vi "GetType.vi"(8 "error in (no error)":errorcluster, 11 "Configure Acceleration Msg":refnum<class "Configure Acceleration Msg.lvclass">) -> (0 "error out":errorcluster, 2 "Data Sample":variant, 3 "Configure Acceleration Msg":refnum<class "Configure Acceleration Msg.lvclass">)   [LabVIEW 2015, in "CS++Motor.lvlib" / "Configure Acceleration Msg.lvclass"]
uses:
  Configure Acceleration Msg.lvclass
  Configure Acceleration Msg.lvclass/Configure Acceleration Msg.ctl
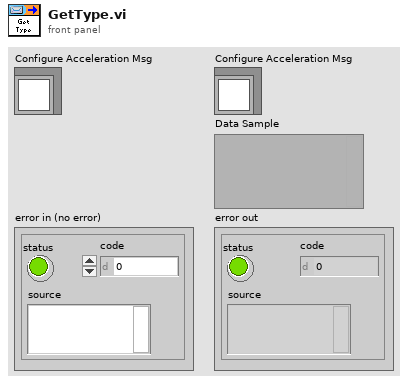
[diagram p1: front panel]
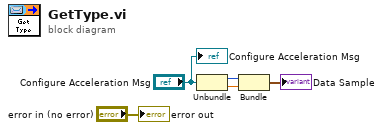
[diagram p0: block diagram]
diagram:
  n1 = Unbundle("Configure Acceleration Msg") -> (w2:u8, w1:dbl)
  n2 = Bundle("AxisNumber"=w2, "Acceleration"=w1) -> (→"Data Sample":cluster{"AxisNumber":u8, "Acceleration":dbl})  [unwired: 1 in]
  "error out" <- "error in (no error)"
  "Configure Acceleration Msg" <- "Configure Acceleration Msg"
